vi "udp_receiver_sample_2.vi"() -> ()   [LabVIEW 2025]
panel:
  out "element":sgl format="%#_6f"
  out "Waveform Graph 5":sgl[](graph)
  out "Waveform Graph 4":sgl[](graph)
  out "Waveform Graph 3":sgl[](graph)
  out "Waveform Graph 2":sgl[](graph)
  out "size(s)":i32
  in  "Boolean 2":bool
  out "Waveform Graph":sgl[](graph)
  in  "Boolean":bool
  out "error out":errorcluster
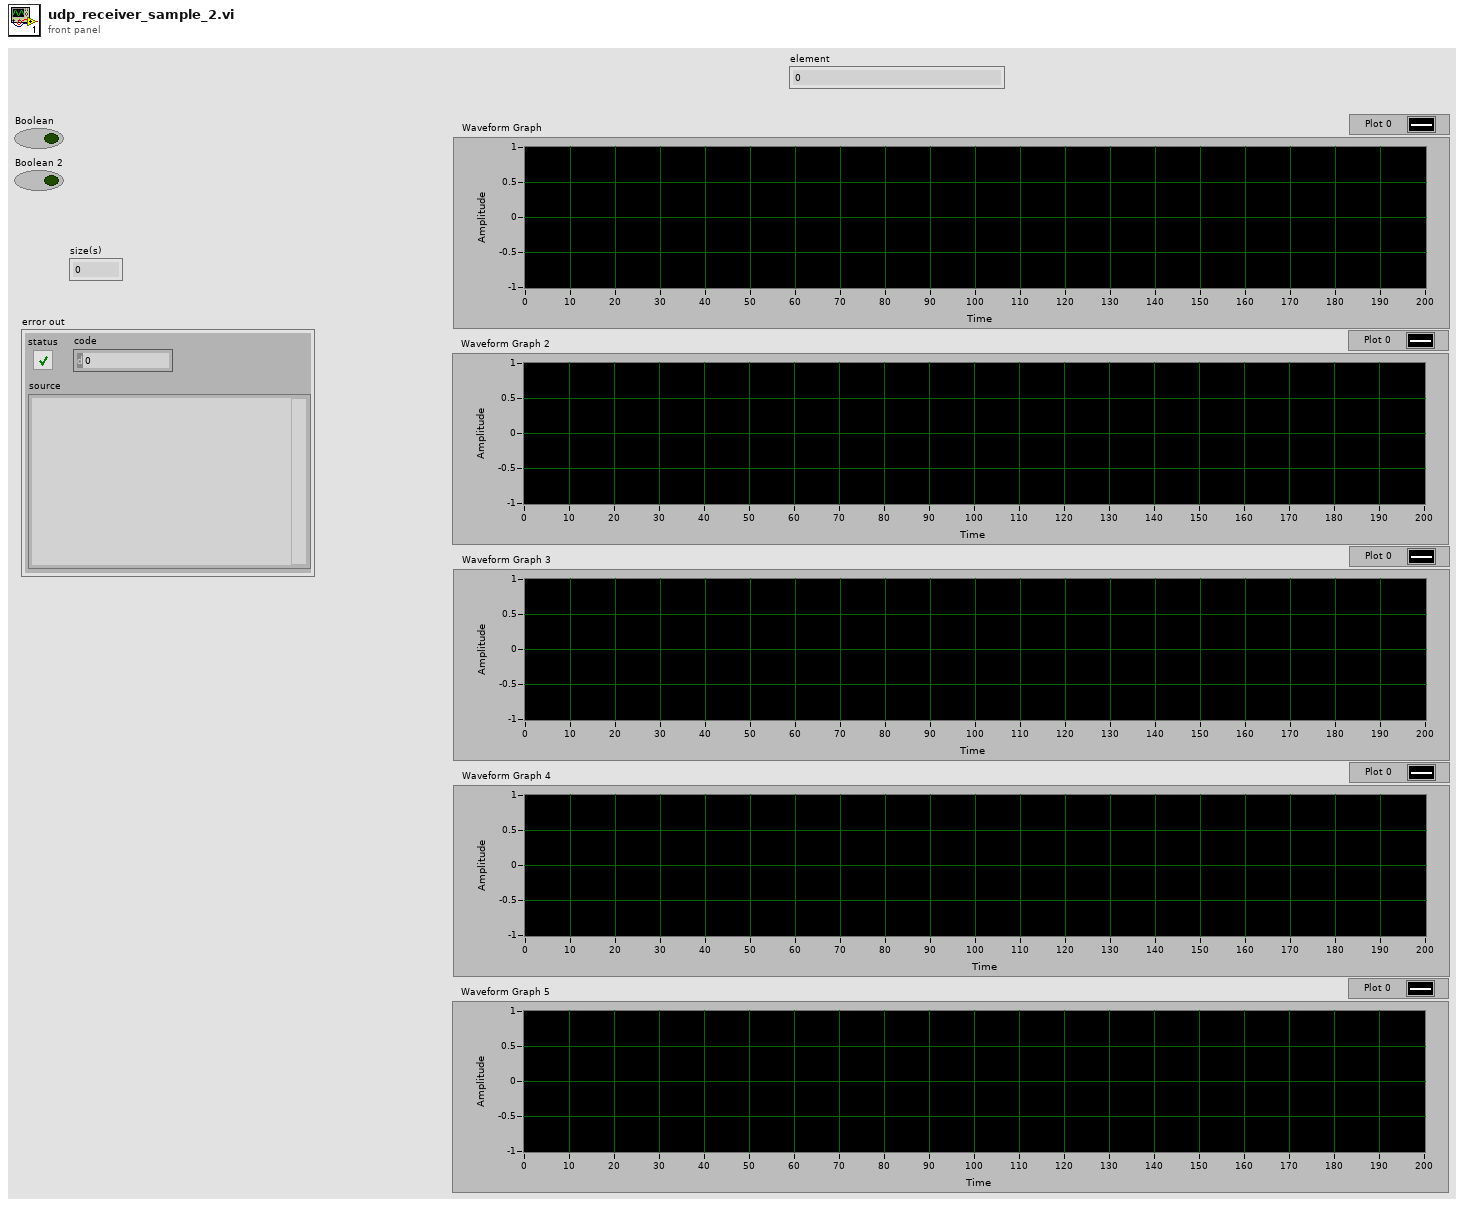
[diagram p1: front panel]
types:
  T1 = enum16{"big-endian, network order", "native, host order", "little-endian"}
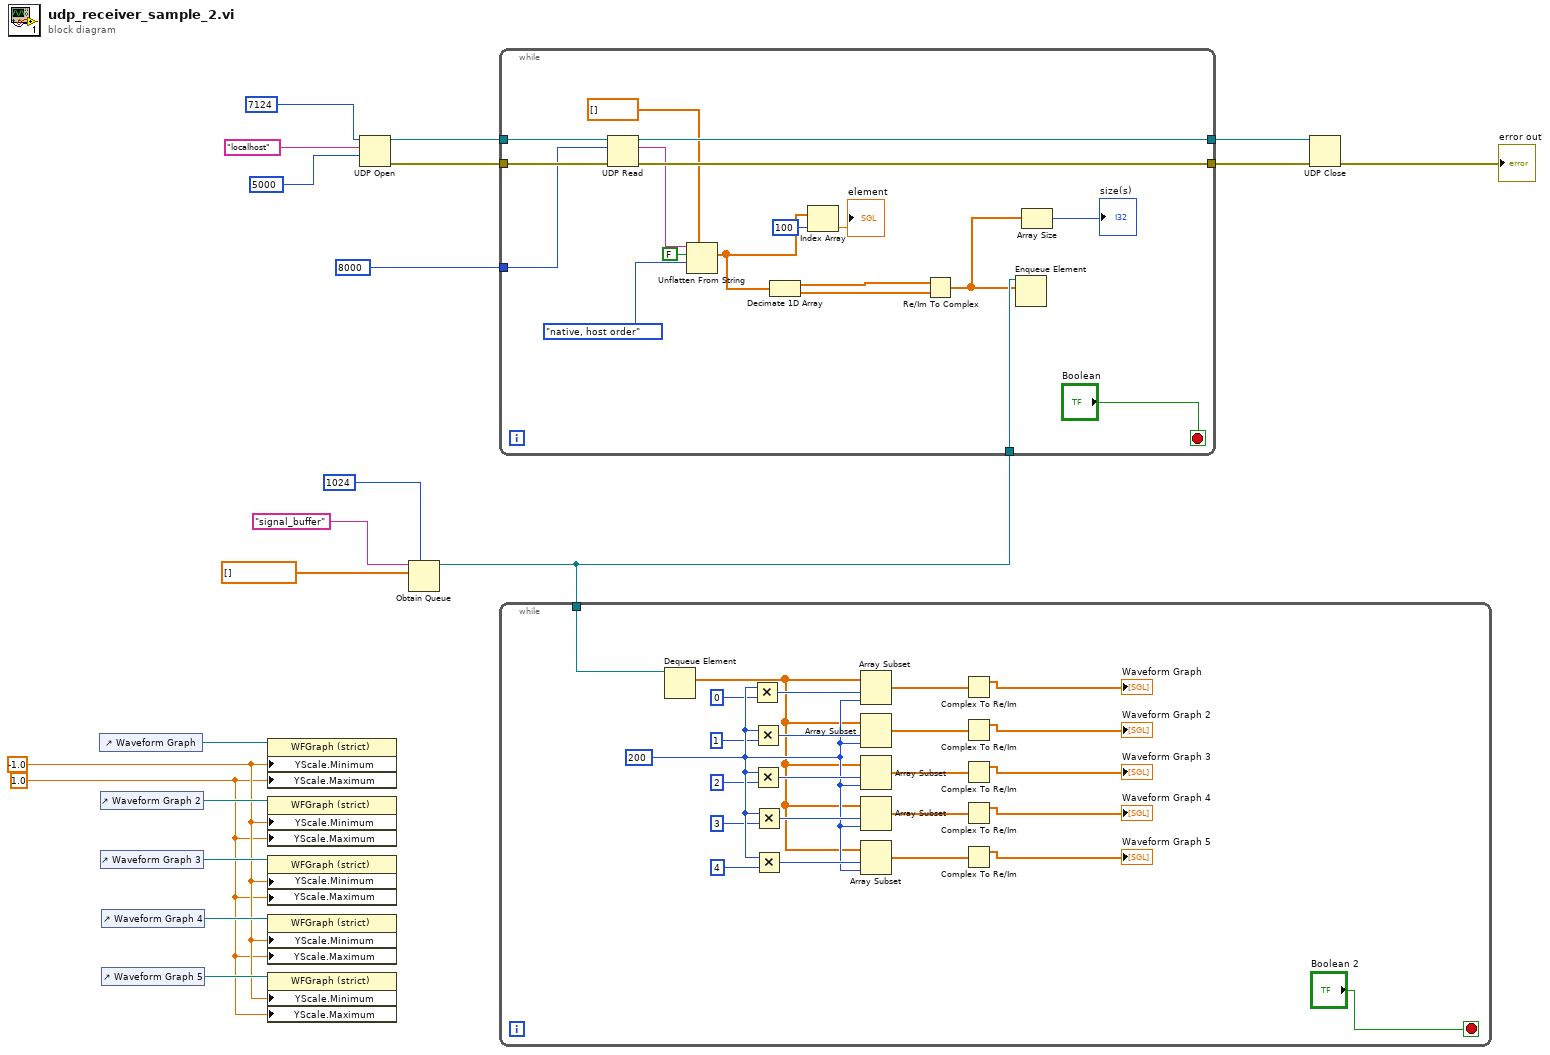
[diagram p0: block diagram]
diagram:
  w1 = 1.0 ("Y Scale.Range:Minimum")
  w2 = -1.0 ("Y Scale.Range:Minimum")
  n1 = control-ref of="Waveform Graph"() -> (w7:refnum<vi>)
  n2 = control-ref of="Waveform Graph 2"() -> (w6:refnum<vi>)
  n3 = control-ref of="Waveform Graph 3"() -> (w5:refnum<vi>)
  n4 = control-ref of="Waveform Graph 4"() -> (w4:refnum<vi>)
  n5 = control-ref of="Waveform Graph 5"() -> (w3:refnum<vi>)
  n6 = property class="WFGraph (strict)"(reference=w7, "YScale.Minimum"=w2, "YScale.Maximum"=w1) -> ()  [unwired: 1 in, 2 out]
  n7 = property class="WFGraph (strict)"(reference=w6, "YScale.Minimum"=w2, "YScale.Maximum"=w1) -> ()  [unwired: 1 in, 2 out]
  n8 = property class="WFGraph (strict)"(reference=w5, "YScale.Minimum"=w2, "YScale.Maximum"=w1) -> ()  [unwired: 1 in, 2 out]
  n9 = property class="WFGraph (strict)"(reference=w4, "YScale.Minimum"=w2, "YScale.Maximum"=w1) -> ()  [unwired: 1 in, 2 out]
  n10 = property class="WFGraph (strict)"(reference=w3, "YScale.Minimum"=w2, "YScale.Maximum"=w1) -> ()  [unwired: 1 in, 2 out]
  n11 = UDP Open(9:5000 ("timeout ms (25000)"), 10:"localhost" ("service name"), 11:u16 7124 ("port")) -> (port=w20:refnum<k16>, 0:w16:errorcluster)  [unwired: 2 in, 1 out]
  n12 = Obtain Queue(max queue size (-1, unlimited)=1024, name (unnamed)="signal_buffer", element data type=csg[] [] ("x + iy")) -> (queue out=w8:refnum<queue>)  [unwired: 2 in, 2 out]
  n13 = while {
    tunnel: w20 -> [w38]
    tunnel: w16 -> [w37]
    tunnel: [w36] -> w15
    tunnel: [w34] -> w14
    tunnel: 8000 ("max size (548)") -> [w33]
    tunnel: w8 -> [w32]
    stop <- "Boolean" stop-if-true
    n14 = UDP Read(connection ID=w38, max size (548)=w33, 8:w37) -> (data out=w23:string, error out=w36:errorcluster, 3:w34:refnum<k16>)  [unwired: 1 in, 2 out]
    n15 = Unflatten From String(type=sgl[] [] ("array"), binary string=w23, data includes array or string size? (T)=FALSE, byte order (0:big-endian, network order)=T1."native, host order") -> (value=w21:sgl[])  [unwired: 1 in, 2 out]
    n16 = Decimate 1D Array(w21) -> (w31:sgl[], w30:sgl[])
    n17 = Index Array(array=w21, index=100) -> (element=→"element":sgl)
    n18 = Re/Im To Complex(1:w30, 2:w31) -> (0:w28:csg[])
    n19 = Enqueue Element(queue=w32, element=w28) -> ()  [unwired: 2 in, 3 out]
    n20 = Array Size(array=w28) -> (size(s)=→"size(s)":i32)
  }
  n21 = while {
    tunnel: w8 -> [w62]
    stop <- "Boolean 2" stop-if-true
    w55 = 200 ("length")
    n22 = Dequeue Element(queue=w62) -> (element=w49:csg[])  [unwired: 2 in, 3 out]
    n23 = Multiply(x=w55, y=0 ("length")) -> (x*y=w60:i32)
    n24 = Multiply(x=w55, y=1 ("length")) -> (x*y=w59:i32)
    n25 = Multiply(x=w55, y=2 ("length")) -> (x*y=w58:i32)
    n26 = Multiply(x=w55, y=3 ("length")) -> (x*y=w57:i32)
    n27 = Multiply(x=w55, y=4 ("length")) -> (x*y=w56:i32)
    n28 = Array Subset(array=w49, index=w60, length=w55) -> (w48:csg[])
    n29 = Array Subset(array=w49, index=w59, length=w55) -> (w47:csg[])
    n30 = Array Subset(array=w49, index=w58, length=w55) -> (w46:csg[])
    n31 = Array Subset(array=w49, index=w57, length=w55) -> (w45:csg[])
    n32 = Array Subset(array=w49, index=w56, length=w55) -> (w44:csg[])
    n33 = Complex To Re/Im(x + iy=w48) -> (x=→"Waveform Graph":sgl[])  [unwired: 1 out]
    n34 = Complex To Re/Im(x + iy=w47) -> (x=→"Waveform Graph 2":sgl[])  [unwired: 1 out]
    n35 = Complex To Re/Im(x + iy=w46) -> (x=→"Waveform Graph 3":sgl[])  [unwired: 1 out]
    n36 = Complex To Re/Im(x + iy=w45) -> (x=→"Waveform Graph 4":sgl[])  [unwired: 1 out]
    n37 = Complex To Re/Im(x + iy=w44) -> (x=→"Waveform Graph 5":sgl[])  [unwired: 1 out]
  }
  n38 = UDP Close(connection ID=w14, 8:w15) -> (error out=→"error out":errorcluster)  [unwired: 1 out]
